vi "SendPulse.vi"(7 "LabVIEW Web Service Request":refnum<class "Web Request.lvclass">) -> (3 "status":string)   [LabVIEW 2017]
uses:
  <vilib>/wsapi/Web Request.lvclass
panel:
  out "permissions":string[](array[string])
  out "groups":string[](array[string])
  out "username":string
  out "key":u8[](array[numeric])
  out "Pulse":variant[](array[variant])
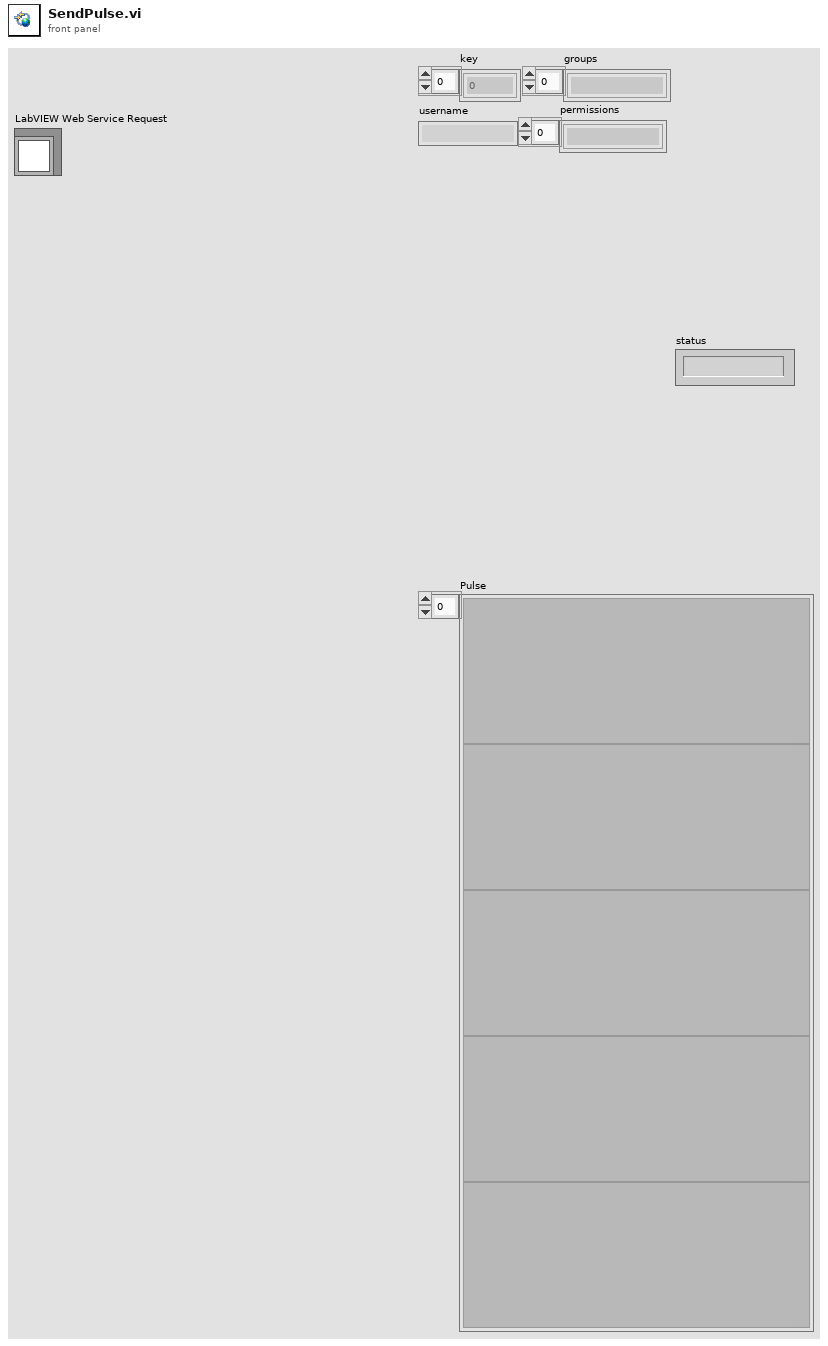
[diagram p1: front panel]
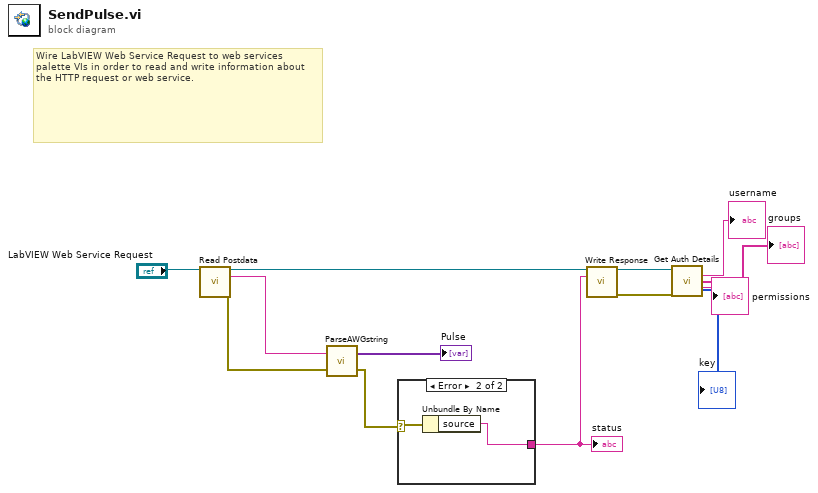
[diagram p0: block diagram]
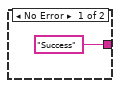
[diagram p2: hidden frame]
diagram:
  # "Wire LabVIEW Web Service Request to web services palette VIs in order to read and write information about the HTTP request or web service."
  n1 = call <vilib>:"Read Postdata.vi"("LabVIEW Web Service Request"="LabVIEW Web Service Request") -> ("LabVIEW Web Service Request out"=w8:refnum<class "Web Request.lvclass">, "postdata"=w10:string, "error out"=w9:errorcluster)  [unwired: 12 in]
  n2 = call "ParseAWGstring.vi"("error constant"=w9, "String"=w10) -> ("error out"=w12:errorcluster, "Array"=→"Pulse":variant[])
  n3 = case shown="Error" w12 {
    selector: w12 -> [_ w16]
    tunnel: ["Success" w15] -> w7
    frame No Error {
    }
    frame Error {
      n4 = Unbundle By Name(w16) -> ("source"=w15:string)
    }
  }
  "status" <- w7
  n5 = call <vilib>:"Write Response.vi"("LabVIEW Web Service Request"=w8, "response string"=w7) -> ("LabVIEW Web Service Request out"=w6:refnum<class "Web Request.lvclass">, "error out"=w5:errorcluster)  [unwired: 12 in]
  n6 = call <vilib>:"Get Auth Details.vi"("LabVIEW Web Service Request"=w6, "error in (no error)"=w5) -> ("username"=→"username":string, "groups"=→"groups":string[], "permissions"=→"permissions":string[], "key"=→"key":u8[])  [unwired: 8 in, 2 out]
